vi "toString.vi"(11 "Telemetry":T1={"SPI"={"SPI_Ack Read"=FALSE, "SPI_Read Flag"=FALSE, "SPI_Read Data"=0, "SPI_Write Data"=0, "SPI_Write Flag"=FALSE, "SPI_Total Bytes"=0, "SPI_Total Bits"=0, "SPI_CS"=0, "SPI_CS Active State"=FALSE, "SPI_Clock Divider"=0, "SPI_CPHA"=FALSE, "SPI_CPOL"=FALSE, "SPI_Cmd"=enum."Idle", "SPI_Port"=0, "SPI_Start"=FALSE, "Ready"=FALSE}, "sbRIO"={"Supply Voltage (V)"=0.0, "FPGA LED"=FALSE, "Chassis Temperature"=0.0}, "Throttles"={"Throttles Consistent?"=FALSE, "Throttles In Range?"=FALSE, "Average Throttle (%)"=0.0, "Throttle 2 (V)"=0.0, "Throttle 2 (%)"=0.0, "Throttle 1 (V)"=0.0, "Throttle 1 (%)"=0.0, "Throttle 2 Max"=0.0, "Throttle 2 Min"=0.0, "Throttle 1 Max"=0.0, "Throttle 1 Min"=0.0}, "Loads & Shutdown"={"RTDS Enable"=FALSE, "TSMS Status"=FALSE, "Positive AIR Enable"=FALSE, "cRIO Shutdown 2"=TRUE, "cRIO Shutdown 1"=TRUE, "Latch Status"=FALSE, "Coolant Pump"=FALSE, "BMS OK"=FALSE, "IMD In"=FALSE, "BSPD In"=FALSE, "Brake Light Out"=FALSE, "Green LED"=enum."Off", "Yellow LED"=enum."Off", "Red LED"=enum."Off"}, "Motor Controller"={"Motor Controller Dash Switch"=FALSE, "Motor Controller Enable"=FALSE}, "Sensors"={"RL Tick Period"=0, "RR Tick Period"=0, "FR Tick Period"=0, "FL Tick Period"=0, "RR Shock (V)"=0.0, "RL Shock (V)"=0.0, "FR Shock (V)"=0.0, "FL Shock (V)"=0.0, "RR Stopped"=FALSE, "RL Stopped"=FALSE, "FR Stopped"=FALSE, "FL Stopped"=FALSE, "Steering Wheel Middle"=0.34827280044555664, "Steering Wheel Angle (degrees)"=0.0, "High Current OK?"=FALSE, "Low Current OK?"=FALSE, "Rear BPS OK?"=TRUE, "Front BPS OK?"=TRUE, "Rear BP (psi)"=185.44775390625, "Front BP (psi)"=186.34033203125, "High Current (A)"=-864.89453125, "Low Current (A)"=-866.732421875}} {"SPI"."SPI_CS" format="%08b"}) -> (3 "String":string)   [LabVIEW 2014]
uses:
  FPGA Telemetry.ctl
  FPGA/SPI/Controls/FPGA SPI_FPGA SPI State.ctl
  Dash LED Status.ctl
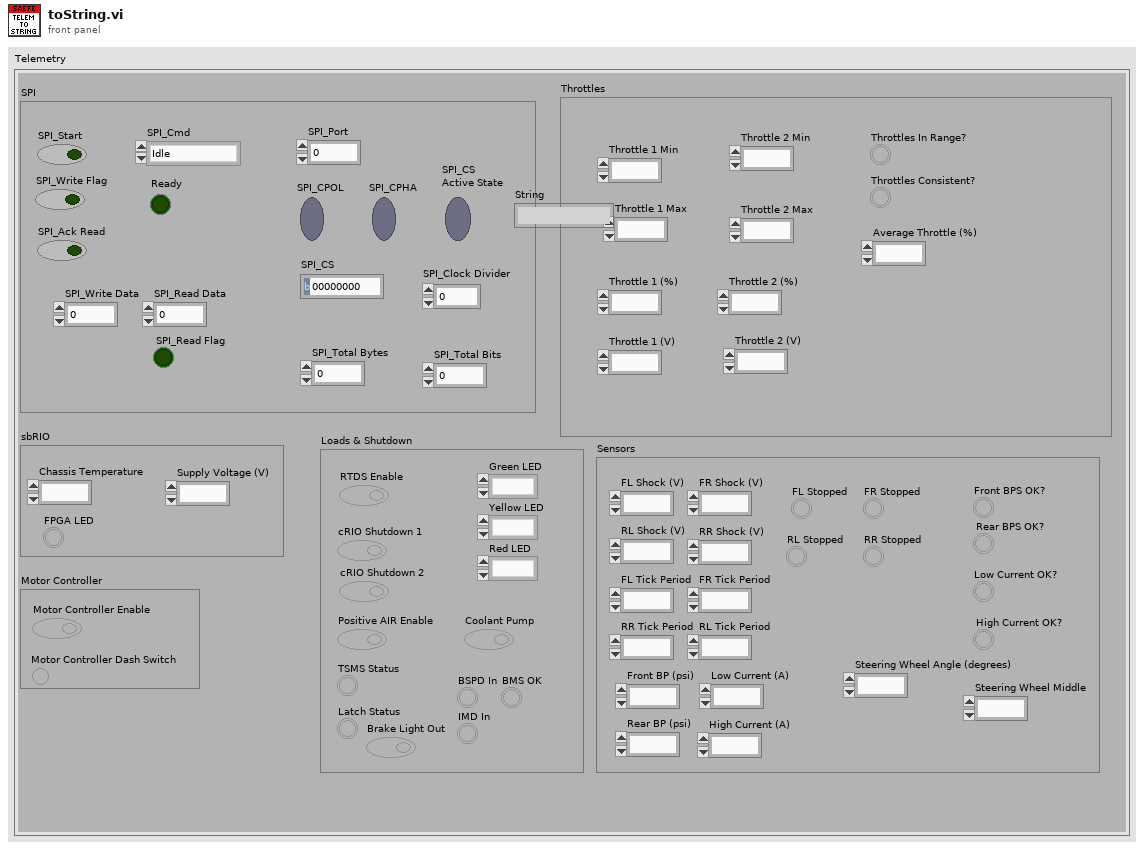
[diagram p1: front panel]
types:
  T1 = typedef "FPGA Telemetry.ctl" = cluster{"SPI":cluster{"SPI_Ack Read":bool, "SPI_Read Flag":bool, "SPI_Read Data":u8, "SPI_Write Data":u8, "SPI_Write Flag":bool, "SPI_Total Bytes":u16, "SPI_Total Bits":u16, "SPI_CS":u8, "SPI_CS Active State":bool, "SPI_Clock Divider":u32, "SPI_CPHA":bool, "SPI_CPOL":bool, "SPI_Cmd":T2, "SPI_Port":i8, "SPI_Start":bool, "Ready":bool}, "sbRIO":cluster{"Supply Voltage (V)":fxp<+/-,25,6>, "FPGA LED":bool, "Chassis Temperature":fxp<+/-,16,9>}, "Throttles":cluster{"Throttles Consistent?":bool, "Throttles In Range?":bool, "Average Throttle (%)":fxp<+/-,29,18>, "Throttle 2 (V)":fxp<+/-,24,5>, "Throttle 2 (%)":fxp<+/-,27,18>, "Throttle 1 (V)":fxp<+/-,24,5>, "Throttle 1 (%)":fxp<+/-,27,18>, "Throttle 2 Max":fxp<+,16,4>, "Throttle 2 Min":fxp<+,16,4>, "Throttle 1 Max":fxp<+,16,4>, "Throttle 1 Min":fxp<+,16,4>}, "Loads & Shutdown":cluster{"RTDS Enable":bool, "TSMS Status":bool, "Positive AIR Enable":bool, "cRIO Shutdown 2":bool, "cRIO Shutdown 1":bool, "Latch Status":bool, "Coolant Pump":bool, "BMS OK":bool, "IMD In":bool, "BSPD In":bool, "Brake Light Out":bool, "Green LED":T3, "Yellow LED":T3, "Red LED":T3}, "Motor Controller":cluster{"Motor Controller Dash Switch":bool, "Motor Controller Enable":bool}, "Sensors":cluster{"RL Tick Period":u32, "RR Tick Period":u32, "FR Tick Period":u32, "FL Tick Period":u32, "RR Shock (V)":fxp<+/-,24,5>, "RL Shock (V)":fxp<+/-,24,5>, "FR Shock (V)":fxp<+/-,24,5>, "FL Shock (V)":fxp<+/-,24,5>, "RR Stopped":bool, "RL Stopped":bool, "FR Stopped":bool, "FL Stopped":bool, "Steering Wheel Middle":fxp<+/-,26,5>, "Steering Wheel Angle (degrees)":fxp<+/-,31,13>, "High Current OK?":bool, "Low Current OK?":bool, "Rear BPS OK?":bool, "Front BPS OK?":bool, "Rear BP (psi)":fxp<+/-,27,16>, "Front BP (psi)":fxp<+/-,27,16>, "High Current (A)":fxp<+/-,24,15>, "Low Current (A)":fxp<+/-,24,15>}}
  T2 = typedef "FPGA SPI_FPGA SPI State.ctl" = enum8{"Idle", "Read/Write SPI", "Configure"}
  T3 = typedef "Dash LED Status.ctl" = enum16{"Off", "Flashing", "On"}
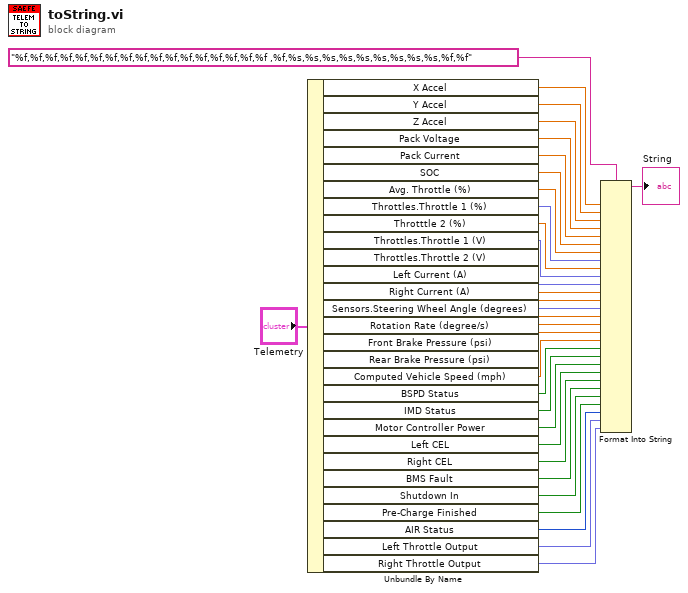
[diagram p0: block diagram]
diagram:
  n1 = Unbundle By Name("Telemetry") -> ("X Accel"=w31:dbl, "Y Accel"=w30:dbl, "Z Accel"=w29:dbl, "Pack Voltage"=w28:dbl, "Pack Current"=w27:dbl, "SOC"=w26:dbl, "Avg. Throttle (%)"=w25:dbl, "Throttles.Throttle 1 (%)"=w24:fxp<+/-,27,18>, "Throtttle 2 (%)"=w23:dbl, "Throttles.Throttle 1 (V)"=w22:fxp<+/-,24,5>, "Throttles.Throttle 2 (V)"=w21:fxp<+/-,24,5>, "Left Current (A)"=w20:dbl, "Right Current (A)"=w19:dbl, "Sensors.Steering Wheel Angle (degrees)"=w18:fxp<+/-,31,13>, "Rotation Rate (degree/s)"=w17:dbl, "Front Brake Pressure (psi)"=w16:dbl, "Rear Brake Pressure (psi)"=w15:dbl, "Computed Vehicle Speed (mph)"=w14:dbl, "BSPD Status"=w13:bool, "IMD Status"=w12:bool, "Motor Controller Power"=w11:bool, "Left CEL"=w10:bool, "Right CEL"=w9:bool, "BMS Fault"=w8:bool, "Shutdown In"=w7:bool, "Pre-Charge Finished"=w6:bool, "AIR Status"=w5:enum16{"Off", "Precharge", "On"}, "Left Throttle Output"=w1:fxp<+/-,20,7>, "Right Throttle Output"=w2:fxp<+/-,20,7>)
  n2 = Format Into String(format string="%f,%f,%f,%f,%f,%f,%f,%f,%f,%f,%f,%f,%f,%f,%f,%f,%f ,%f,%s,%s,%s,%s,%s,%s,%s,%s,%s,%f,%f", w31, w30, w29, w28, w27, w26, w25, w24, w23, w22, w21, w20, w19, w18, w17, w16, w15, w14, w13, w12, w11, w10, w9, w8, w7, w6, w5, w1, w2) -> (resulting string=→"String":string)  [unwired: 2 in, 1 out]
